vi "Sub_element_Matrix.vi"(1 "Length of Beam":dbl, 3 "Young's Modulus":dbl, 4 "No. of Nodes":i32, 5 "Height":dbl, 7 "Width":dbl, 10 "Density":dbl) -> (17 "Element Length":dbl, 18 "M Element Matrix":dbl[][](array[numeric]), 19 "K Element Matrix":dbl[][](array[numeric]))   [LabVIEW 2021]
panel:
  in  "Accelerometer Mass":dbl
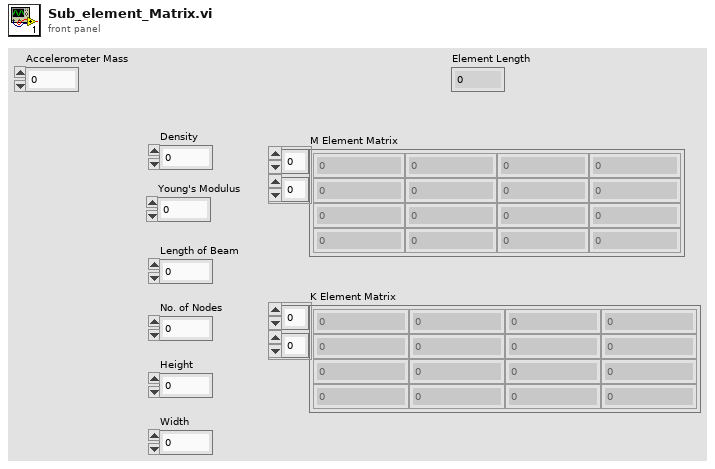
[diagram p1: front panel]
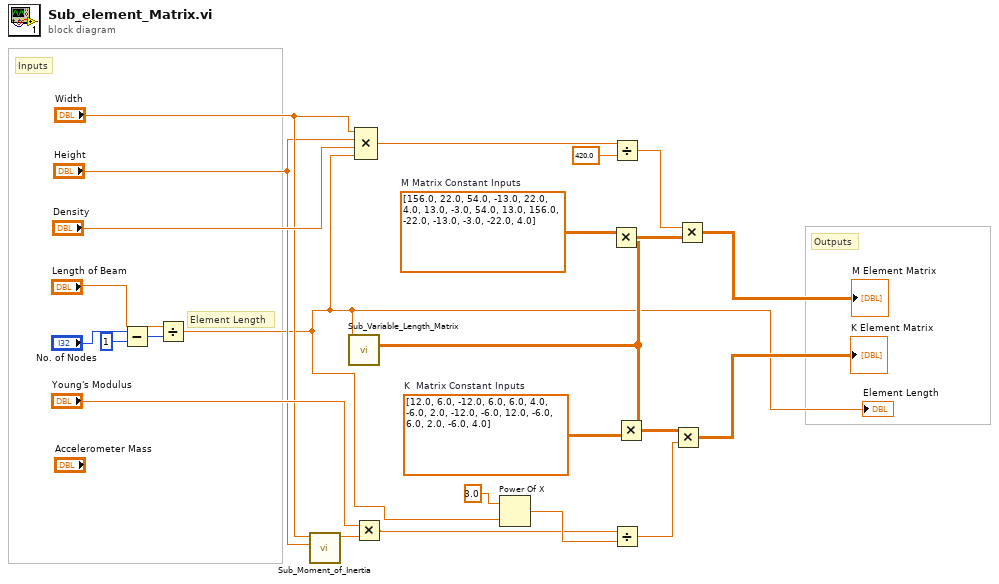
[diagram p0: block diagram]
diagram:
  w13 = dbl[][] [[12.0, 6.0, -12.0, 6.0], [6.0, 4.0, -6.0, 2.0], [-12.0, -6.0, 12.0, -6.0], [6.0, 2.0, -6.0, 4.0]]  # K  Matrix Constant Inputs
  w20 = dbl[][] [[156.0, 22.0, 54.0, -13.0], [22.0, 4.0, 13.0, -3.0], [54.0, 13.0, 156.0, -22.0], [-13.0, -3.0, -22.0, 4.0]]  # M Matrix Constant Inputs
  # "Outputs"
  # "Element Length"
  # "Inputs"
  n1 = Subtract(x="No. of Nodes", y=1) -> (x-y=w19:i32)
  n2 = Divide(x="Length of Beam", y=w19) -> (x/y=w2:dbl)
  "Element Length" <- w2
  n3 = call "Sub_Moment_of_Inertia.vi"("Height"="Height", "Width"="Width") -> ("Numeric"=w4:dbl)  [unwired: 9 in]
  n4 = call "Sub_Variable_Length_Matrix.vi"("Numeric"=w2) -> ("Array"=w14:dbl[][])  [unwired: 10 in]
  n5 = Multiply(x="Young's Modulus", y=w4) -> (x*y=w7:dbl)
  n6 = Compound Arithmetic op=MULTIPLY("Width", "Height", "Density", w2) -> (w22:dbl)
  n7 = Power Of X(1:w2, 2:3.0 ("x")) -> (0:w12:dbl)
  n8 = Multiply(x=w20, y=w14) -> (x*y=w23:dbl[][])
  n9 = Divide(x=w22, y=420.0) -> (x/y=w24:dbl)
  n10 = Divide(x=w7, y=w12) -> (x/y=w11:dbl)
  n11 = Multiply(x=w14, y=w13) -> (x*y=w10:dbl[][])
  n12 = Multiply(x=w10, y=w11) -> (x*y=→"K Element Matrix":dbl[][])
  n13 = Multiply(x=w24, y=w23) -> (x*y=→"M Element Matrix":dbl[][])
